vi "Query Capabilities (Temperature).vi"(0 "VISA resource name":refnum<visa-resource-name>, 5 "Absolute Maximums (T)":bool=TRUE, 11 "error in (no error)":errorcluster) -> (4 "VISA resource name out":refnum<visa-resource-name>, 6 "Maximum Temperature":dbl max=12.0 step=1.0, 15 "error out":errorcluster)   [LabVIEW 2020, in "NH Research Regenerative Test Series.lvlib"]
doc: "This query will retrieve the absolute maximum temperature setting for the Module. Returns -1 if temperature is not available."
uses:
  NH Research Regenerative Test Series.lvlib
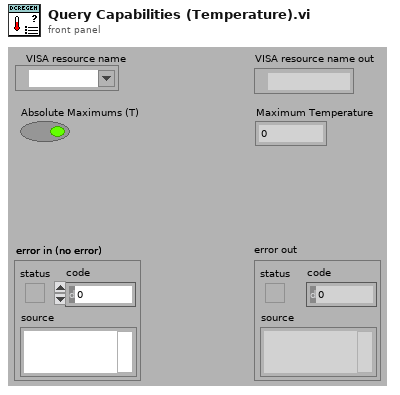
[diagram p1: front panel]
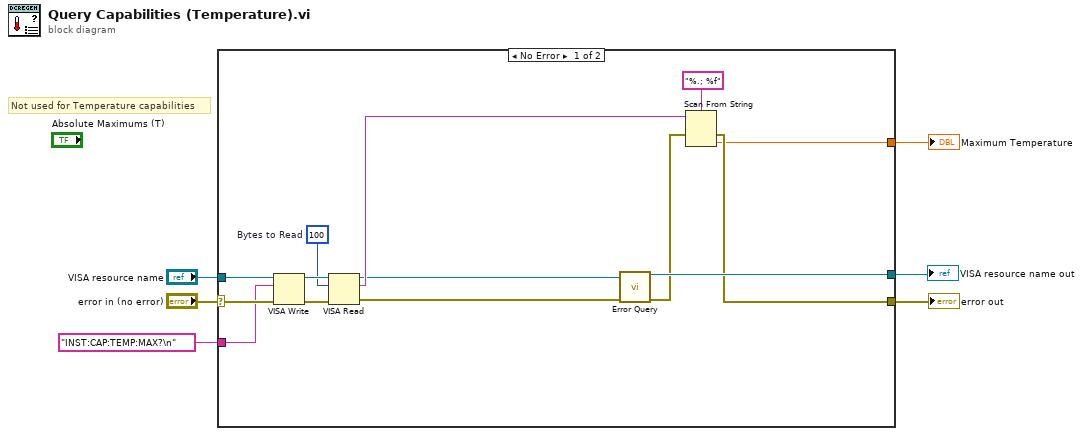
[diagram p0: block diagram]
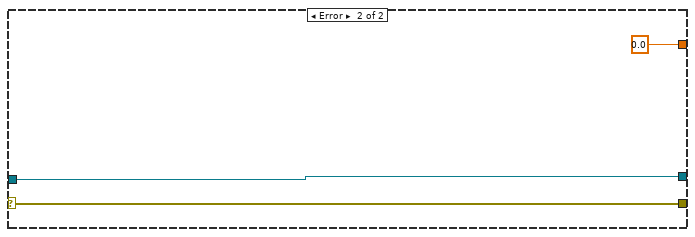
[diagram p2: hidden frame]
diagram:
  # "Not used for Temperature capabilities"
  n1 = case shown="No Error" "error in (no error)" {
    selector: "error in (no error)" -> [w18 w23]
    tunnel: [w10 w23] -> w5
    tunnel: [w16 w22] -> w3
    tunnel: "VISA resource name" -> [w17 w22]
    tunnel: [w7 0.0] -> w2
    tunnel: "INST:CAP:TEMP:MAX?\n" ("write buffer") -> [w14 _]
    frame No Error {
      w13 = u32 100  # Bytes to Read
      n2 = VISA Write(VISA resource name=w17, write buffer=w14, error in (no error)=w18) -> (VISA resource name out=w19:refnum<visa-resource-name>, error out=w20:errorcluster)  [unwired: 1 out]
      n3 = VISA Read(VISA resource name=w19, byte count=w13, error in (no error)=w20) -> (VISA resource name out=w9:refnum<visa-resource-name>, read buffer=w11:string, error out=w8:errorcluster)  [unwired: 1 out]
      n4 = call "Error Query.vi"("VISA resource name"=w9, "error in (no error)"=w8) -> ("VISA resource name out"=w16:refnum<visa-resource-name>, "error out"=w15:errorcluster)  [unwired: 10 in, 2 out]
      n5 = Scan From String(format string="%.; %f", input string=w11, error in=w15) -> (error out=w10:errorcluster, output 1=w7:dbl)  [unwired: 2 in, 2 out]
    }
    frame Error {
    }
  }
  "error out" <- w5
  "VISA resource name out" <- w3
  "Maximum Temperature" <- w2
